vi "Request Channel Names Async.vi"(7 "Source ID":u32, 10 "Group":refnum<class "Group.lvclass">, 11 "Discovery":refnum<class "NodeDiscovery.lvclass">) -> ()   [LabVIEW 2020, in "Vecto.lvlib" / "RemoteDataService.lvclass"]
uses:
  RemoteDataService.lvclass
  RemoteDataService.lvclass/RemoteDataService.ctl
  NodeDiscovery/NodeDiscovery.lvclass
  proto/ServiceType/Enumeration.ctl
  proto/ServiceType/ServiceType.lvlib
  Vecto.lvlib
  <vilib>/httpClient/LabVIEWHTTPClient.lvlib
  Publish Config.ctl
  Publish Config Response Group.ctl
  Publish Config Response.ctl
  Group/Group.lvclass
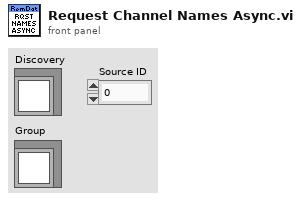
[diagram p1: front panel]
types:
  T1 = typedef "ServiceType.lvlib/Enumeration.ctl" = enum16{"SERVICETYPE_UNKNOWN", "SERVICETYPE_TCPSERVER", "SERVICETYPE_HTTPSERVER"}
  T2 = typedef "Vecto.lvlib/Publish Config Response.ctl" = cluster{"Groups":T3[]}
  T3 = typedef "Vecto.lvlib/Publish Config Response Group.ctl" = cluster{"Name":string, "Endpoint":T4, "Channels":string[], "OwningTask":string}
  T4 = typedef "Vecto.lvlib/Publish Config.ctl" = cluster{"Address":string, "Port":u16}
  T5 = typedef "Discovery.lvlib/Data.ctl" = cluster{"node_id":u32, "name":string, "ip":u32, "status":string, "services":T6[], "system":string, "cluster":string}
  T6 = typedef "Service.lvlib/Data.ctl" = cluster{"type":T1, "port":i32}
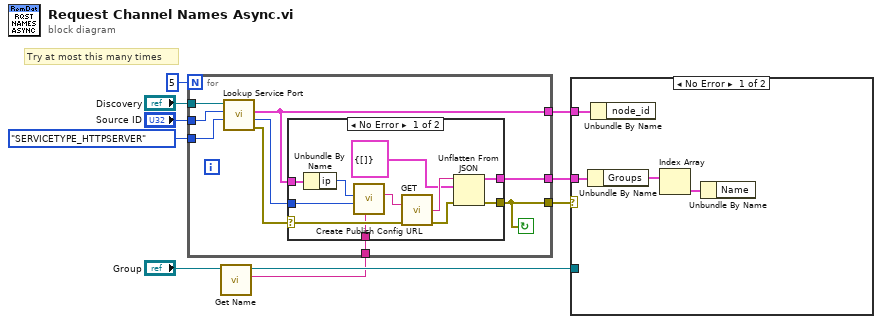
[diagram p0: block diagram]
diagram:
  # "Try at most this many times"
  n1 = call "Get Name.vi"("Group in"="Group") -> ("Name"=w1:string, "Group out"=w2:refnum<class "Group.lvclass">)  [unwired: 8 in, 1 out]
  n2 = for {
    N: 5 -> [_]
    tunnel: Enumeration."SERVICETYPE_HTTPSERVER" ("Service Type") -> [w19]
    tunnel: "Source ID" -> [w18]
    tunnel: "Discovery" -> [w17]
    tunnel: [w14] -> w6
    tunnel: [w13] -> w5
    tunnel: [w12] -> w4
    tunnel: w1 -> [w11]
    stop <- w12 continue-if-true
    n3 = call "Lookup Service Port.vi"("Service Type"=w19, "node_id"=w18, "NodeDiscovery in"=w17) -> ("error out"=w16:errorcluster, "port"=w15:i32, "Node"=w14:T5)  [unwired: 5 in, 1 out]
    n4 = case shown="No Error" w16 {
      selector: w16 -> [w26 w31]
      tunnel: w15 -> [w28 _]
      tunnel: w14 -> [w30 _]
      tunnel: [w22 _] -> w13
      tunnel: [w21 w31] -> w12
      tunnel: w11 -> [w20 _]
      frame No Error {
        n5 = Unbundle By Name(w30) -> ("ip"=w29:u32)
        n6 = call "Create Publish Config URL.vi"("Group (All)"=w20, "port"=w28, "ip"=w29) -> ("String"=w27:string)  [unwired: 8 in]
        n7 = call <vilib>:"GET.vi"("url"=w27, "error in (no error)"=w26) -> ("body"=w25:string, "error out"=w23:errorcluster)  [unwired: 10 in, 2 out]
        n8 = Unflatten From JSON(JSON string=w25, type and defaults=T2 {"Groups"=[]} ("Publish Config Response"), error in (no error)=w23) -> (value=w22:T2, error out=w21:errorcluster)  [unwired: 4 in]
      }
      frame Error {
      }
    }
  }
  n9 = case shown="No Error" w4 {
    tunnel: w6 -> [w35 _]
    tunnel: w5 -> [w34 _]
    tunnel: w2 -> [_ _]
    frame No Error {
      n10 = Unbundle By Name(w34) -> ("Groups"=w33:T3[])
      n11 = Unbundle By Name(w35) -> ()  [unwired: 1 out]
      n12 = Index Array(array=w33) -> (element=w32:T3)  [unwired: 1 in]
      n13 = Unbundle By Name(w32) -> ()  [unwired: 1 out]
    }
    frame Error {
    }
  }
